vi "mod_exponential average.vi"(9 "reset?":bool, 10 "N":dbl format="%.2f", 11 "in":dbl format="%.2f") -> (3 "out":dbl format="%.2f")   [LabVIEW 2020, in "niAMT.lvlib"]
uses:
  <vilib>/addons/Modulation/niAMT.lvlib
panel:
  # "out = (1/N)(out(n-1) + in*(N-1))"
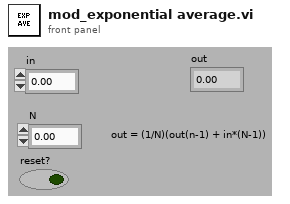
[diagram p1: front panel]
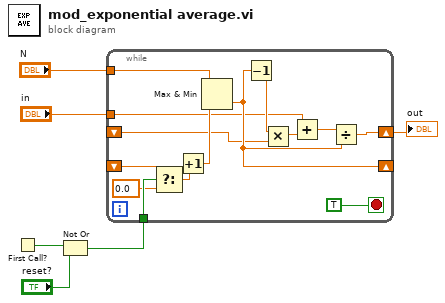
[diagram p0: block diagram]
diagram:
  n1 = First Call?() -> (First Call?: T/F=w6:bool)
  n2 = Not Or(1:"reset?", 2:w6) -> (0:w2:bool)
  n3 = while {
    shift-right: [w15] -> w3
    shift-left: _ -> [w8]
    shift-right: [w12] -> _
    shift-left: _ -> [w18]
    tunnel: "N" -> [w13]
    tunnel: w2 -> [w19]
    tunnel: "in" -> [w7]
    stop <- TRUE stop-if-true
    n4 = Select(t=w18, s=w19, f=0.0) -> (s? t:f=w17:dbl)
    n5 = Increment(x=w17) -> (x+1=w14:dbl)
    n6 = Max & Min(x=w13, y=w14) -> (min(x,y)=w12:dbl)  [unwired: 1 out]
    n7 = Decrement(x=w12) -> (x-1=w9:dbl)
    n8 = Multiply(x=w9, y=w8) -> (x*y=w10:dbl)
    n9 = Add(x=w7, y=w10) -> (x+y=w20:dbl)
    n10 = Divide(x=w20, y=w12) -> (x/y=w15:dbl)
  }
  "out" <- w3
